vi "EMS Set Device Parameter Status.vi"(4 "error":string, 6 "Status":T1, 8 "error in (no error)":errorcluster, 9 "Parameter Name":string, 10 "IED Name":string, 11 "Master Controller in":refnum<class "Master Controller.lvclass">) -> (0 "error out":errorcluster, 3 "Master Controller out":refnum<class "Master Controller.lvclass">)   [LabVIEW 2015, in "Master Controller Core.lvlib" / "Master Controller.lvclass"]
uses:
  Master Controller.lvclass
  SCADA Core/SCADA Abstract Messages/Set Device Parameter Status Msg/Set Device Parameter Status.ctl
  Communications/SCADA Communcations Actor/SCADA Communications/Controls/EMS Message Cluster.ctl
  Master Controller.lvclass/Master Controller.ctl
  Communications/SCADA Communcations Actor/SCADA Communications Messages/Transmit EMS Message Msg/Transmit EMS Message Msg.lvclass/Transmit EMS Message Msg.ctl
  <vilib>/ActorFramework/Message Enqueuer/Message Enqueuer.lvclass/Message Enqueuer.ctl
  <vilib>/ActorFramework/Message Enqueuer/Enqueue.vi
  <vilib>/ActorFramework/Message Priority Queue/Priority Enqueue.vi
  Communications/SCADA Communcations Actor/SCADA Communications Messages/Transmit EMS Message Msg/Transmit EMS Message Msg.lvclass
  Utilities/Message Strings.llb/Message String Utilities.lvlib
  Communications/SCADA Communcations Actor/SCADA Communications/SCADA Communications.lvclass
  SCADA Core/SCADA Abstract Messages/Set Device Parameter Status Msg/Set Device Parameter Status Msg.lvclass
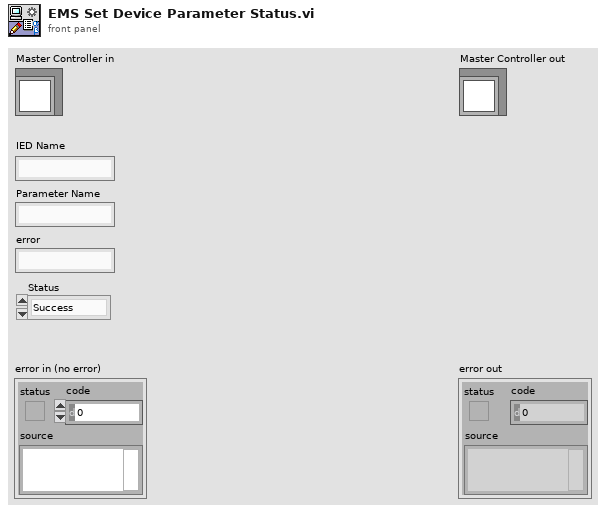
[diagram p1: front panel]
types:
  T1 = typedef "SCADA Core.lvlib/Set Device Parameter Status Msg.lvclass/Set Device Parameter Status.ctl" = enum16{"Success", "Failure"}
  T2 = typedef "SCADA Communcations Actor.lvlib/SCADA Communications.lvclass/EMS Message Cluster.ctl" = cluster{"Name":string, "Content":string}
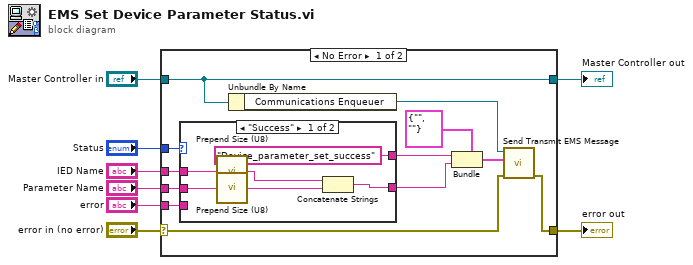
[diagram p0: block diagram]
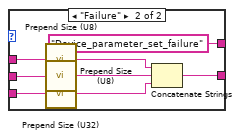
[diagram p2: hidden frame]
diagram:
  n1 = case shown="No Error" "error in (no error)" {
    selector: "error in (no error)" -> [w14 w36]
    tunnel: [w9 w36] -> w7
    tunnel: [w15 w35] -> w5
    tunnel: "Master Controller in" -> [w15 w35]
    tunnel: "Status" -> [w13 _]
    tunnel: "IED Name" -> [w12 _]
    tunnel: "Parameter Name" -> [w11 _]
    tunnel: "error" -> [w10 _]
    frame No Error {
      n2 = case shown="\"Success\"" w13 {
        tunnel: ["Device_parameter_set_success" ("Name") "Device_parameter_set_failure" ("Name")] -> w19
        tunnel: w10 -> [_ w32]
        tunnel: w11 -> [w25 w33]
        tunnel: w12 -> [w24 w31]
        tunnel: [w21 w27] -> w20
        frame "Success" {
          n3 = call "Prepend Size (U8).vi"("String in"=w24) -> ("String out"=w23:string)
          n4 = call "Prepend Size (U8).vi"("String in"=w25) -> ("String out"=w22:string)
          n5 = Concatenate Strings(w23, w22) -> (w21:string)
        }
        frame "Failure" {
          n6 = call "Prepend Size (U8).vi"("String in"=w31) -> ("String out"=w29:string)
          n7 = call "Prepend Size (U8).vi"("String in"=w33) -> ("String out"=w30:string)
          n8 = call "Prepend Size (U32).vi"("String in"=w32) -> ("String out"=w28:string)
          n9 = Concatenate Strings(w29, w30, w28) -> (w27:string)
        }
      }
      n10 = Unbundle By Name(w15) -> ("Communications Enqueuer"=w17:refnum<class "Message Enqueuer.lvclass">)
      n11 = Bundle(cluster=T2 {"Name"="", "Content"=""} ("Message"), "Name"=w19, "Content"=w20) -> (w18:T2)
      n12 = call "Send Transmit EMS Message.vi"("error in (no error)"=w14, "Message"=w18, "Message Enqueuer"=w17) -> ("error out"=w9:errorcluster)  [unwired: 7 in, 1 out]
    }
    frame Error {
    }
  }
  "error out" <- w7
  "Master Controller out" <- w5
